vi "Create Stop Event.vi"(8 "error in (no error)":errorcluster, 11 "Results in":refnum<class "Results.lvclass">) -> (0 "error out":errorcluster, 2 "stop event":refnum<user-event>, 3 "Results out":refnum<class "Results.lvclass">)   [LabVIEW 2015, in "Result Actor.lvlib" / "Results.lvclass"]
uses:
  Results.lvclass
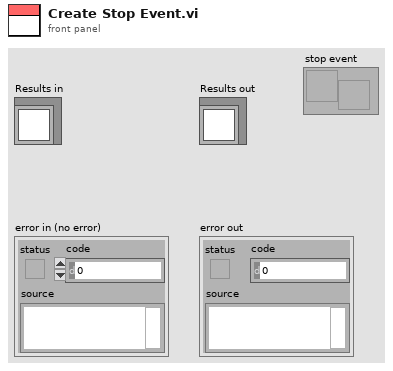
[diagram p1: front panel]
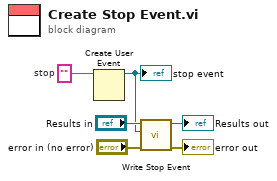
[diagram p0: block diagram]
diagram:
  w2 = ""  # stop
  n1 = Create User Event(user event datatype=w2) -> (user event=w1:refnum<user-event>)  [unwired: 1 in, 1 out]
  "stop event" <- w1
  n2 = call "Write Stop Event.vi"("error in (no error)"="error in (no error)", "stop event"=w1, "Results in"="Results in") -> ("error out"=→"error out":errorcluster, "Results out"=→"Results out":refnum<class "Results.lvclass">)  [unwired: 7 in]
